vi "Read Multiple String.vi"(8 "error in (no error)":errorcluster, 10 "Char/Str":bool, 11 "Tags":string) -> (0 "error out":errorcluster, 2 "Data Byte":string[](array[string]), 3 "Siemens Ctr out":T1)   [LabVIEW 2014]
uses:
  Simatic S7.lvlib
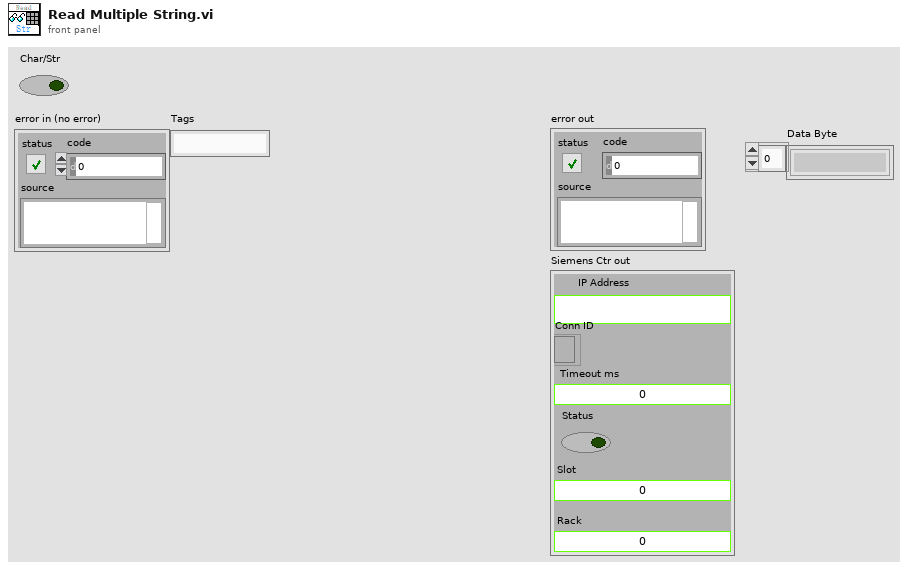
[diagram p1: front panel]
types:
  T1 = typedef "Simatic S7.lvlib/Siemens Ref.ctl" = cluster{"IP Address ":string, "Conn ID":refnum<k5>, "Timeout ms":i32, "Status":bool, "Slot":u16, "Rack":u16}
  T2 = typedef "Simatic S7.lvlib/Operation Siemens Ref.ctl" = enum16{"Init", "Add Ref", "Get Ref", "Set Error", "Close Close"}
  T3 = typedef "PLC Address.ctl" = cluster{"Address Areas":u8, "Data Type":enum8{"Bit", "Byte", "int", "Word", "Dint", "Dword", "Real", "String"}, "DB.No":u16, "Byte":u32, "Length":u16, "Item":u16}
  T4 = typedef "Semaphore RefNum" = refnum<k1>
  T5 = typedef "Simatic S7.lvlib/Op ip address.ctl" = enum16{"Init", "Add IP", "Get IP"}
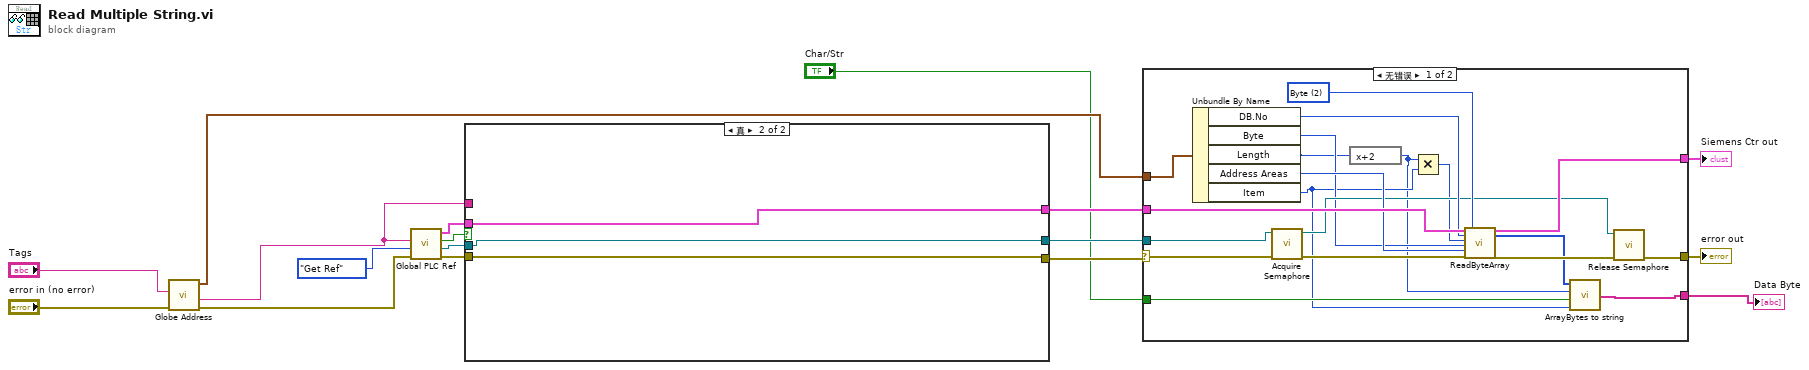
[diagram p0: block diagram]
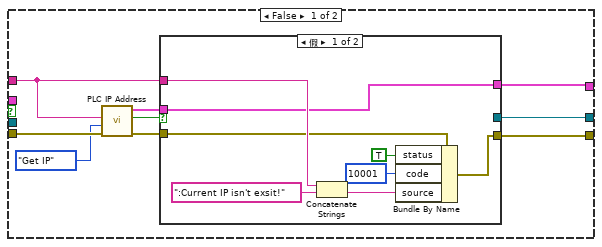
[diagram p3: hidden frame]
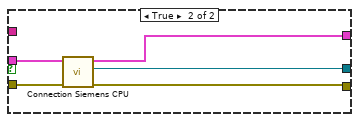
[diagram p4: hidden frame]
diagram:
  n1 = call "Globe Address.vi"("error in (no error)"="error in (no error)", "Tag"="Tags") -> ("error out"=w8:errorcluster, "IP"=w7:string, "ddress"=w5:T3)  [unwired: 6 in, 1 out]
  n2 = call "Global PLC Ref.vi"("error in (no error)"=w8, "Operation Siemens Ref"=Operation_Siemens_Ref."Get Ref", "IP Address"=w7) -> ("error out"=w15:errorcluster, "semaphore"=w13:T4, "Boolean"=w16:bool, "Siemens Ctr out"=w14:T1)  [unwired: 4 in, 1 out]
  n3 = case shown="真" w16 {
    tunnel: w15 -> [w26 w42]
    tunnel: w7 -> [w22 _]
    tunnel: [w20 w42] -> w12
    tunnel: [w19 w40] -> w11
    tunnel: [w18 w41] -> w10
    tunnel: w14 -> [_ w41]
    tunnel: w13 -> [_ w40]
    frame False {
      n4 = call "PLC IP Address.vi"("error in (no error)"=w26, "Operationip"=Op_ip_address."Get IP", "IP Address"=w22) -> ("error out"=w23:errorcluster, "Boolean"=w24:bool, "Siemens Ctr out"=w21:T1)  [unwired: 6 in]
      n5 = case shown="假" w24 {
        tunnel: w23 -> [w32 w39]
        tunnel: w22 -> [w33 _]
        tunnel: w21 -> [w27 w38]
        tunnel: [w28 w37] -> w20
        tunnel: [_ w36] -> w19
        tunnel: [w27 w35] -> w18
        frame False {
          n6 = Concatenate Strings(w33, ":Current IP isn't exsit!") -> (w30:string)
          n7 = Bundle By Name(cluster=w32, "status"=TRUE, "code"=10001, "source"=w30) -> (w28:errorcluster)
        }
        frame True {
          n8 = call "Connection Siemens CPU.vi"("error in (no error)"=w39, "Siemens Ctr in"=w38) -> ("error out"=w37:errorcluster, "semaphore"=w36:T4, "Siemens Ctr out"=w35:T1)  [unwired: 7 in]
        }
      }
    }
    frame True {
    }
  }
  n9 = case shown="无错误" w12 {
    selector: w12 -> [w62 w64]
    tunnel: w11 -> [w56 _]
    tunnel: w10 -> [w60 w63]
    tunnel: w5 -> [w59 _]
    tunnel: [w52 w64] -> w4
    tunnel: [w54 w63] -> w3
    tunnel: "Char/Str" -> [w48 _]
    tunnel: [w46 _] -> w1
    frame No Error {
      w58 = u8 2 items=["Boolen"=1, "Byte"=2] ("Bit/Byte")
      n10 = Unbundle By Name(w59) -> ("DB.No"=w57:u16, "Byte"=w50:u32, "Length"=w44:u16, "Address Areas"=w55:u8, "Item"=w45:u16)
      n11 = call <vilib>:"Acquire Semaphore.vi"("error in (no error)"=w62, "semaphore"=w56) -> ("error out"=w61:errorcluster, "semaphore out"=w51:T4)  [unwired: 3 in, 1 out]
      n12 = expression code="x+2"(w44) -> (w43:u16)
      n13 = Multiply(x=w43, y=w45) -> (x*y=w47:u16)
      n14 = call "ReadByteArray.vi"("Siemens Ctr"=w60, "# DB No."=w57, "#items"=w47, "Item offset [byte]"=w50, "Address Areas"=w55, "error in (no error)"=w61, "Bit/Byte"=w58) -> ("Siemens Ctr out"=w54:T1, "Byte Array"=w49:u8[], "error out"=w53:errorcluster)  [unwired: 10 in]
      n15 = call "ArrayBytes to string.vi"("Array Bytes"=w49, "Sigle length+2"=w43, "Char/Str"=w48, "item"=w45) -> ("String"=w46:string[])  [unwired: 1 in]
      n16 = call <vilib>:"Release Semaphore.vi"("error in (no error)"=w53, "semaphore"=w51) -> ("error out"=w52:errorcluster)  [unwired: 4 in, 1 out]
    }
    frame Error {
    }
  }
  "error out" <- w4
  "Siemens Ctr out" <- w3
  "Data Byte" <- w1
